vi "Hysteresis.vi"(0 "Input":dbl format="%.2p", 5 "level":dbl format="%.2p", 7 "hysteresis":dbl format="%.2p", 9 "type":enum16{"Percentage", "level"}(ring), 11 "error in (no error)":errorcluster) -> (8 "ACT_Dv_too_large":bool, 15 "error out":errorcluster)   [LabVIEW 2022 SP3]
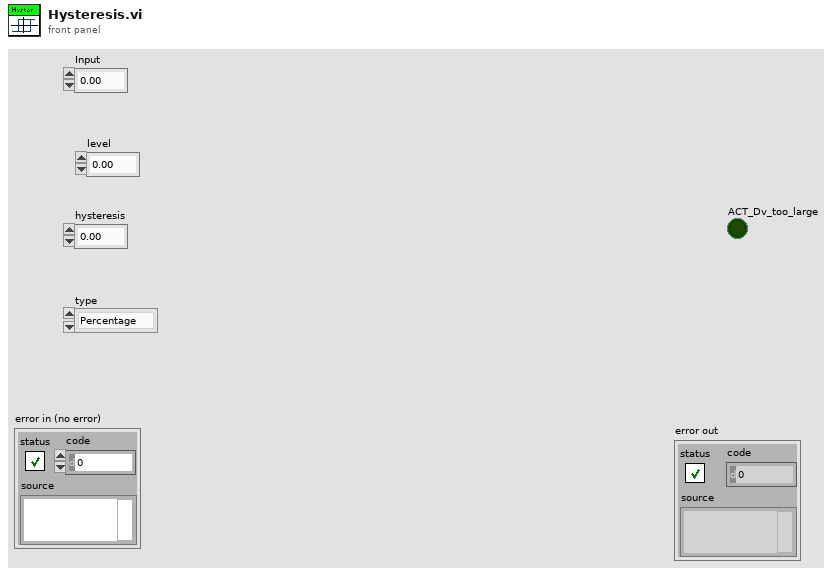
[diagram p1: front panel]
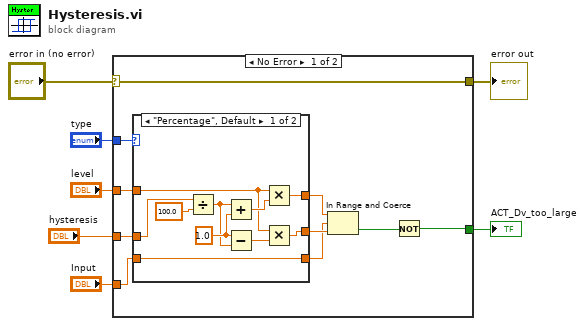
[diagram p0: block diagram]
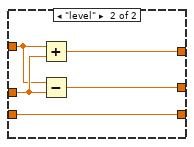
[diagram p2: hidden frame]
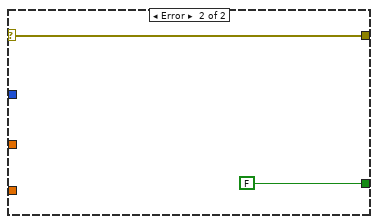
[diagram p3: hidden frame]
diagram:
  n1 = case shown="No Error" "error in (no error)" {
    selector: "error in (no error)" -> [w11 w34]
    tunnel: [w11 w34] -> w6
    tunnel: [w8 FALSE ("trigger detected?")] -> w5
    tunnel: "Input" -> [w15 _]
    tunnel: "hysteresis" -> [w16 _]
    tunnel: "type" -> [w17 _]
    tunnel: "level" -> [w10 _]
    frame No Error {
      n2 = case shown="\"Percentage\", Default" w17 {
        tunnel: w16 -> [w27 w31]
        tunnel: w15 -> [w19 w29]
        tunnel: [w21 w32] -> w14
        tunnel: [w20 w30] -> w13
        tunnel: [w19 w29] -> w12
        tunnel: w10 -> [w18 w28]
        frame "Percentage", Default {
          w25 = 1.0 ("y")
          n3 = Divide(x=w27, y=100.0) -> (x/y=w24:dbl)
          n4 = Add(x=w24, y=w25) -> (x+y=w23:dbl)
          n5 = Subtract(x=w25, y=w24) -> (x-y=w22:dbl)
          n6 = Multiply(x=w18, y=w23) -> (x*y=w21:dbl)
          n7 = Multiply(x=w18, y=w22) -> (x*y=w20:dbl)
        }
        frame "level" {
          n8 = Add(x=w28, y=w31) -> (x+y=w32:dbl)
          n9 = Subtract(x=w28, y=w31) -> (x-y=w30:dbl)
        }
      }
      n10 = In Range and Coerce(upper limit=w14, x=w12, lower limit=w13) -> (In Range?=w9:bool)  [unwired: 1 out]
      n11 = Not(x=w9) -> (.not. x?=w8:bool)
    }
    frame Error {
    }
  }
  "error out" <- w6
  "ACT_Dv_too_large" <- w5
